vi "Update Numeric Value.vi"(10 "Tree Tag":string, 11 "UI Data In":refnum<class "Settings UI.lvclass">) -> (2 "New Tree Value":string, 3 "UI Data out":refnum<class "Settings UI.lvclass">)   [LabVIEW 2024, in "Output Sequencer.lvlib" / "Settings UI.lvclass"]
uses:
  Settings UI.lvclass
  Settings UI.lvclass/Settings UI.ctl
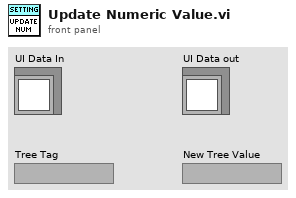
[diagram p1: front panel]
types:
  T1 = typedef "Output Sequencer.lvlib/Settings UI.lvclass/Tree Index Enum.ctl" = enum16{"General Settings", "Num Steps", "Num Analog", "Num Digital", "Show Confirmation", "Interp Priority", "Adv Timing", "Enable Conditions", "Seq Execution", "Reset Test Start", "Only When Test", "Delay After Test", "Start condition", "Re-triggering", "Stop condition", "Stop After Cycles", "Stop Values", "Default Values", "Default Analog", "Default Digital", "Steps", "Step #", "Description", "Precondition", "Duration", "Mode", "Delay Between Vals", "Analog Values", "Digital Values", "Postcondition", "On True", "On False"}
  T2 = typedef "Output Sequencer.lvlib/Settings UI.lvclass/Step Settings.ctl" = cluster{"Description":string, "Precondition":string, "Duration":dbl, "Mode":string, "Delay Between Values":dbl, "Analog Values":string[], "Digital Values":string[], "Postcondition":string, "On True":string, "On False":string}
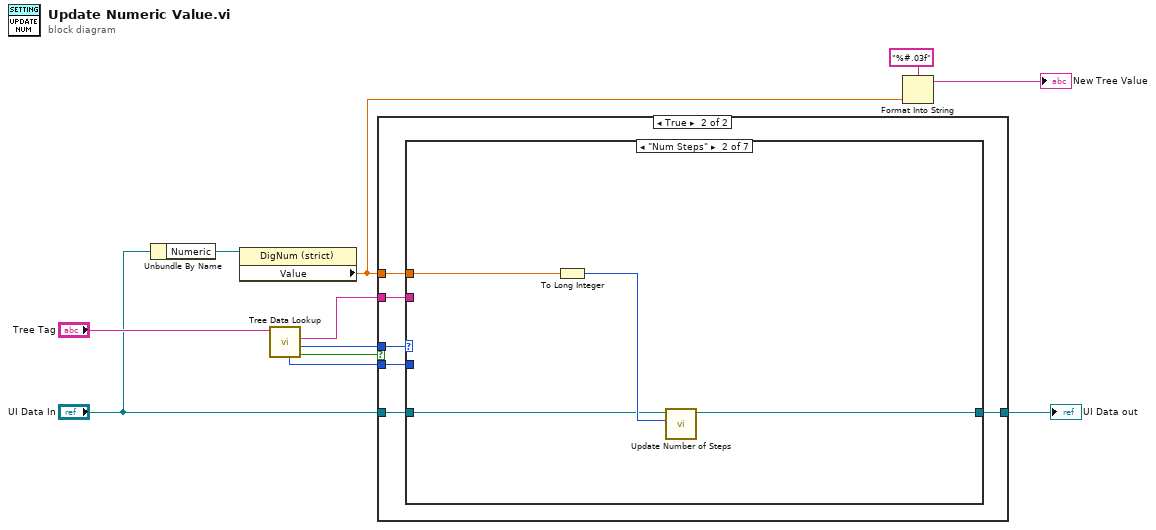
[diagram p0: block diagram]
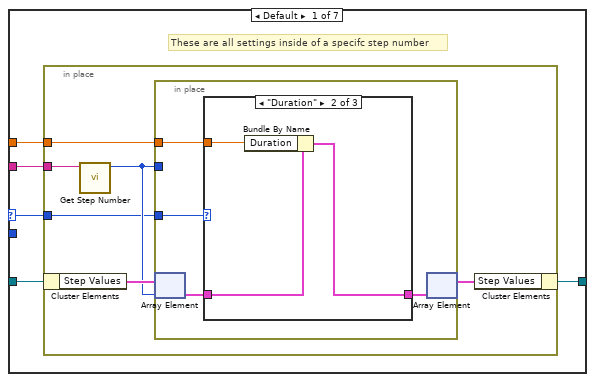
[diagram p3: hidden frame]
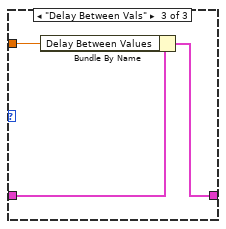
[diagram p5: hidden frame]
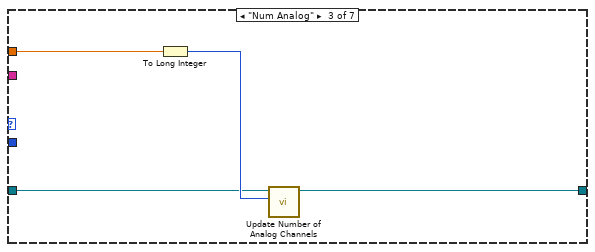
[diagram p6: hidden frame]
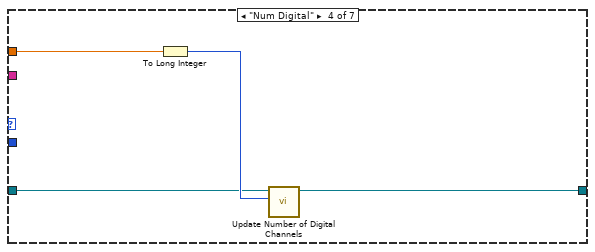
[diagram p7: hidden frame]
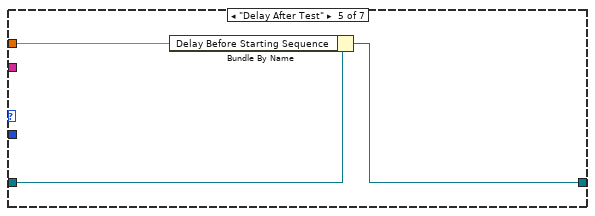
[diagram p8: hidden frame]
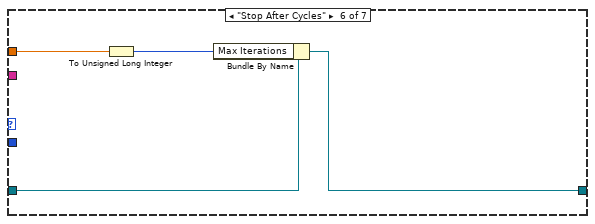
[diagram p9: hidden frame]
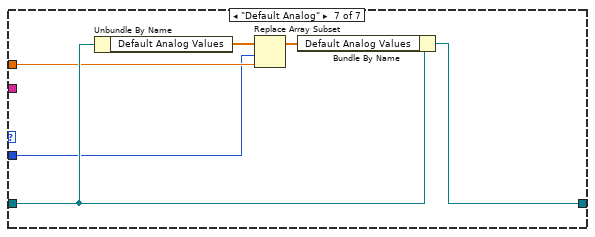
[diagram p10: hidden frame]
diagram:
  n1 = Unbundle By Name("UI Data In") -> ("Numeric"=w8:refnum<vi>)
  n2 = property class="DigNum (strict)"(reference=w8) -> ("Value"=w6:dbl)  [unwired: 1 in, 2 out]
  n3 = call "Tree Data Lookup.vi"("Tag in"="Tree Tag") -> ("Found?"=w4:bool, "Tree Index Enum"=w3:T1, "Tag out"=w5:string, "Item Number"=w2:i32)  [unwired: 5 in, 2 out]
  n4 = case shown="True" w4 {
    tunnel: w6 -> [_ w18]
    tunnel: "UI Data In" -> [w12 w17]
    tunnel: [w12 w16] -> w10
    tunnel: w5 -> [_ w15]
    tunnel: w3 -> [_ w14]
    tunnel: w2 -> [_ w13]
    frame False {
    }
    frame True {
      n5 = case shown="\"Num Steps\"" w14 {
        selector: w14 -> [w19 _ _ _ _ _ _]
        tunnel: w18 -> [w23 w44 w48 w52 w53 w57 w61]
        tunnel: w17 -> [w22 w41 w45 w49 w55 w59 w63]
        tunnel: [w20 w42 w47 w51 w54 w58 w62] -> w16
        tunnel: w15 -> [w21 _ _ _ _ _ _]
        tunnel: w13 -> [_ _ _ _ _ _ w60]
        frame Default {
          # "These are all settings inside of a specifc step number"
          n6 = in-place {
            in-place-border: w23 -> [w29]
            in-place-border: w21 -> [w28]
            in-place-border: w19 -> [w24]
            n7 = in-place-cluster #1(w22) -> ("Step Values"=w27:T2[])
            n8 = call "Get Step Number.vi"("Tree Tag"=w28) -> ("Step Number"=w26:i32)  [unwired: 8 in, 2 out]
            n9 = in-place {
              in-place-border: w29 -> [w33]
              in-place-border: w26 -> [_]
              in-place-border: w24 -> [w30]
              n10 = in-place-array #2(w27, w26) -> (w32:T2)
              n11 = case shown="\"Duration\"" w30 {
                tunnel: w32 -> [w34 w37 w40]
                tunnel: w33 -> [_ w36 w39]
                tunnel: [w34 w35 w38] -> w31
                frame Default {
                }
                frame "Duration" {
                  n12 = Bundle By Name(cluster=w37, "Duration"=w36) -> (w35:T2)
                }
                frame "Delay Between Vals" {
                  n13 = Bundle By Name(cluster=w40, "Delay Between Values"=w39) -> (w38:T2)
                }
              }
              n14 = in-place-array #2(w31) -> (w25:T2[])  [unwired: 1 out]
            }
            n15 = in-place-cluster #1("Step Values"=w25) -> (w20:refnum<class "Settings UI.lvclass">)
          }
        }
        frame "Num Steps" {
          n16 = To Long Integer(number=w44) -> (32bit integer=w43:i32)
          n17 = call "Update Number of Steps.vi"("New Number of Steps"=w43, "UI Data in"=w41) -> ("UI Data in"=w42:refnum<class "Settings UI.lvclass">)  [unwired: 9 in]
        }
        frame "Num Analog" {
          n18 = To Long Integer(number=w48) -> (32bit integer=w46:i32)
          n19 = call "Update Number of Analog Channels.vi"("New Number"=w46, "UI Data in"=w45) -> ("UI Data out"=w47:refnum<class "Settings UI.lvclass">)  [unwired: 9 in]
        }
        frame "Num Digital" {
          n20 = To Long Integer(number=w52) -> (32bit integer=w50:i32)
          n21 = call "Update Number of Digital Channels.vi"("New Number"=w50, "UI Data in"=w49) -> ("UI Data out"=w51:refnum<class "Settings UI.lvclass">)  [unwired: 9 in]
        }
        frame "Delay After Test" {
          n22 = Bundle By Name(cluster=w55, "Delay Before Starting Sequence"=w53) -> (w54:refnum<class "Settings UI.lvclass">)
        }
        frame "Stop After Cycles" {
          n23 = To Unsigned Long Integer(number=w57) -> (unsigned 32bit integer=w56:u32)
          n24 = Bundle By Name(cluster=w59, "Max Iterations"=w56) -> (w58:refnum<class "Settings UI.lvclass">)
        }
        frame "Default Analog" {
          n25 = Unbundle By Name(w63) -> ("Default Analog Values"=w65:dbl[])
          n26 = Replace Array Subset(array=w65, new element=w61, index=w60) -> (w64:dbl[])
          n27 = Bundle By Name(cluster=w63, "Default Analog Values"=w64) -> (w62:refnum<class "Settings UI.lvclass">)
        }
      }
    }
  }
  "UI Data out" <- w10
  n28 = Format Into String(format string="%#.03f", w6) -> (resulting string=→"New Tree Value":string)  [unwired: 2 in, 1 out]
